vi "Experiment header-Interface module.vi"(4 "New Value":dbl, 6 "Name of parameter to update":string, 7 "Header file type":T7=enum."Params for funct acq w ROI or mscn", 8 "error in (no error)":errorcluster, 9 "All header parameters in":T1={"Imaging Protocol"=enum."AOL Z-Stack", "Number of POI"=0, "Number of Miniscans"=0, "Number of Trials"=0, "Number of Cycles "=0, "# Averaged Frames"=0, "Laser power (%)"=0, "Pockels"=0.0, "Acquisition Length (sec)"=0.0, "Fill time (us)"=0.0, "POI Dwell time (us)"=0.0, "Miniscan Dwell time per pixel (us)"=0.0, "PMT 1"=0.0, "PMT 2"=0.0, "Back Apperture"=0.0, "Zoom"=0.0, "Frame Size"=0, "Center Frequency"=0.0, "Field of View"=0.0, "DwellTime (us)"=0.0, "Wavelength (nm)"=0.0, "AOL Z"=0.0, "AOL Mode"=enum."Raster", "GridXY"=0.0, "GridZ"=0.0, "TriggerDelay (sec)"=0.0, "Number of Pixels in Miniscan"=0, "Experiment folder path"=path "", "X centre"=0.0, "Y centre"=0.0, "Angle (degrees)"=0.0, "Plane Mode"=0, "Software version"=0.0, "Objective"="Olympus  20X", "MotorZ Calibration"=0, "Pockels Calibration"=0, "Threshold"=[], "Video length (sec)"=0.0, "Frame rate (fps)"=0, "Rectangle ROI length (pixels)"=0, "Rectangle ROI height (pixels)"=0} {"Pockels" format="%#.6g"; "Software version" format="%#.6g"; "Plane Mode" items=["XY Plane"]; "Angle (degrees)" format="%#.6g"; "Frame Size" items=["100X100"=100, "128X128"=128, "200X200"=200, "256X256"=256, "512X512"=512, "1024x1024"=1024, "2048x2048"=2048]; "Back Apperture" format="%#.6g"; "PMT 2" format="%#.6g"; "PMT 1" format="%#.6g"; "Miniscan Dwell time per pixel (us)" format="%#.6g"; "Zoom" format="%#.6g"; "POI Dwell time (us)" format="%#.6g"; "Acquisition Length (sec)" format="%#.6g"; "Fill time (us)" format="%#.6g"}, 10 "Function":T8, 11 "Experiment data folder path":path) -> (0 "error out":errorcluster, 1 "All header parameters out":T1={"Imaging Protocol"=enum."AOL Z-Stack", "Number of POI"=0, "Number of Miniscans"=0, "Number of Trials"=0, "Number of Cycles "=0, "# Averaged Frames"=0, "Laser power (%)"=0, "Pockels"=0.0, "Acquisition Length (sec)"=0.0, "Fill time (us)"=0.0, "POI Dwell time (us)"=0.0, "Miniscan Dwell time per pixel (us)"=0.0, "PMT 1"=0.0, "PMT 2"=0.0, "Back Apperture"=0.0, "Zoom"=0.0, "Frame Size"=0, "Center Frequency"=0.0, "Field of View"=0.0, "DwellTime (us)"=0.0, "Wavelength (nm)"=0.0, "AOL Z"=0.0, "AOL Mode"=enum."Raster", "GridXY"=0.0, "GridZ"=0.0, "TriggerDelay (sec)"=0.0, "Number of Pixels in Miniscan"=0, "Experiment folder path"=path "", "X centre"=0.0, "Y centre"=0.0, "Angle (degrees)"=0.0, "Plane Mode"=0, "Software version"=0.0, "Objective"="Olympus  20X", "MotorZ Calibration"=0, "Pockels Calibration"=0, "Threshold"=[], "Video length (sec)"=0.0, "Frame rate (fps)"=0, "Rectangle ROI length (pixels)"=0, "Rectangle ROI height (pixels)"=0} {"Pockels" format="%#.6g"; "Software version" format="%#.6g"; "Plane Mode" items=["XY Plane"]; "Angle (degrees)" format="%#.6g"; "Frame Size" items=["100X100"=100, "128X128"=128, "200X200"=200, "256X256"=256, "512X512"=512, "1024x1024"=1024, "2048x2048"=2048]; "Back Apperture" format="%#.6g"; "PMT 2" format="%#.6g"; "PMT 1" format="%#.6g"; "Miniscan Dwell time per pixel (us)" format="%#.6g"; "Zoom" format="%#.6g"; "POI Dwell time (us)" format="%#.6g"; "Acquisition Length (sec)" format="%#.6g"; "Fill time (us)" format="%#.6g"})   [LabVIEW 2013]
uses:
  Typedefs/Header parameters cluster-ALL.ctl
  Typedefs/Imaging Protocols enum.ctl
  Typedefs/Frame Size.ctl
  Typedefs/AOL modes.ctl
  Typedefs/Plane Mode.ctl
  Typedefs/Objective selector control enum.ctl
  Typedefs/Header file interface module functions enum.ctl
  Typedefs/Header file type enum.ctl
  Typedefs/Save-Load-Save as-Load last enum.ctl
panel:
  in  "All params (internal)":T1={"Imaging Protocol"=enum."AOL Z-Stack", "Number of POI"=0, "Number of Miniscans"=0, "Number of Trials"=0, "Number of Cycles "=0, "# Averaged Frames"=0, "Laser power (%)"=0, "Pockels"=0.0, "Acquisition Length (sec)"=0.0, "Fill time (us)"=0.0, "POI Dwell time (us)"=0.0, "Miniscan Dwell time per pixel (us)"=0.0, "PMT 1"=0.0, "PMT 2"=0.0, "Back Apperture"=0.0, "Zoom"=0.0, "Frame Size"=0, "Center Frequency"=0.0, "Field of View"=0.0, "DwellTime (us)"=0.0, "Wavelength (nm)"=0.0, "AOL Z"=0.0, "AOL Mode"=enum."Raster", "GridXY"=0.0, "GridZ"=0.0, "TriggerDelay (sec)"=0.0, "Number of Pixels in Miniscan"=0, "Experiment folder path"=path "", "X centre"=0.0, "Y centre"=0.0, "Angle (degrees)"=0.0, "Plane Mode"=0, "Software version"=0.0, "Objective"="Olympus  20X", "MotorZ Calibration"=0, "Pockels Calibration"=0, "Threshold"=[], "Video length (sec)"=0.0, "Frame rate (fps)"=0, "Rectangle ROI length (pixels)"=0, "Rectangle ROI height (pixels)"=0} {"Pockels" format="%#.6g"; "Software version" format="%#.6g"; "Plane Mode" items=["XY Plane"]; "Angle (degrees)" format="%#.6g"; "Frame Size" items=["100X100"=100, "128X128"=128, "200X200"=200, "256X256"=256, "512X512"=512, "1024x1024"=1024, "2048x2048"=2048]; "Back Apperture" format="%#.6g"; "PMT 2" format="%#.6g"; "PMT 1" format="%#.6g"; "Miniscan Dwell time per pixel (us)" format="%#.6g"; "Zoom" format="%#.6g"; "POI Dwell time (us)" format="%#.6g"; "Acquisition Length (sec)" format="%#.6g"; "Fill time (us)" format="%#.6g"}
  # "Used with the \"Update specific value in memory\" function only"
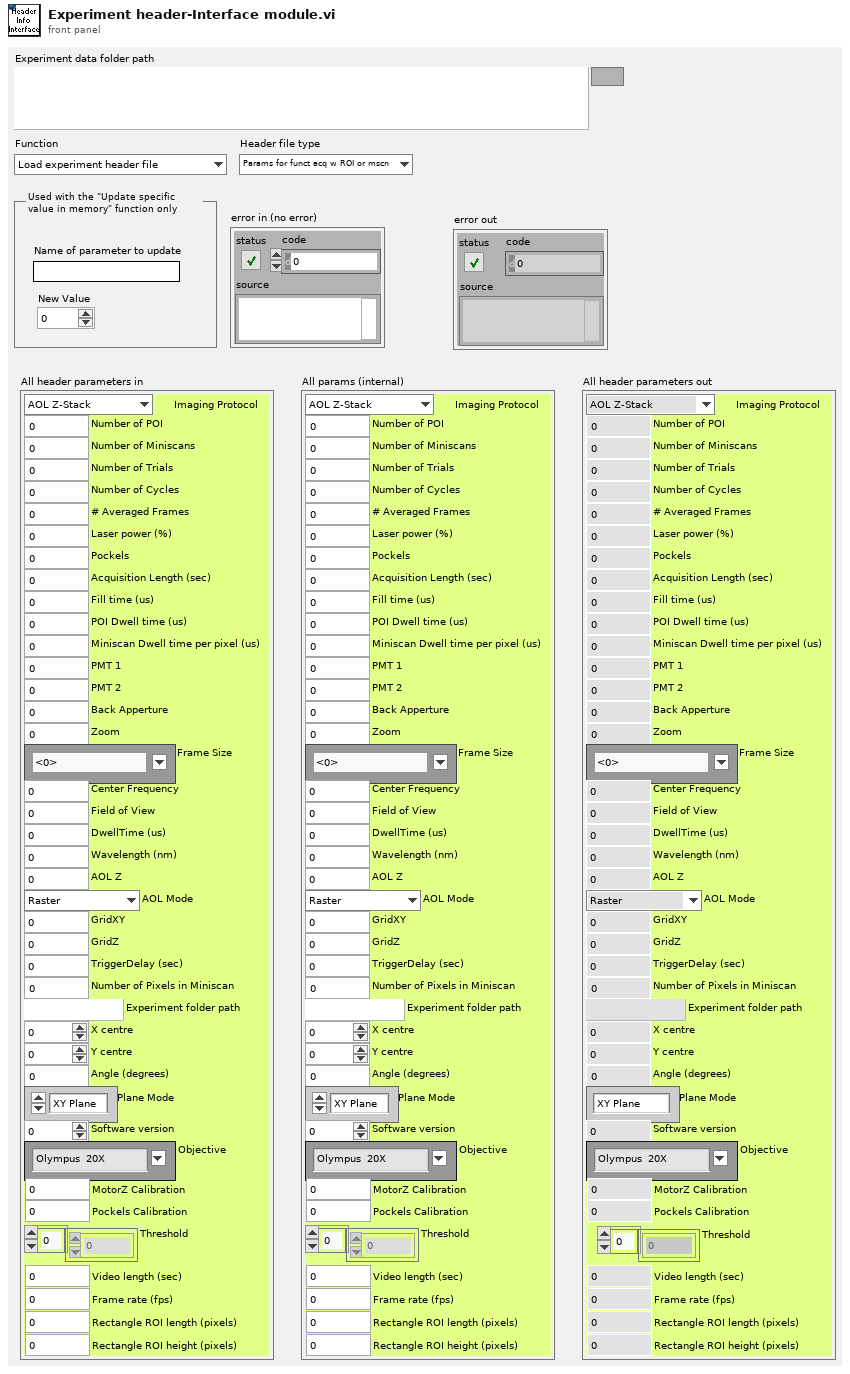
[diagram p1: front panel]
types:
  T1 = typedef "Header parameters cluster-ALL.ctl" = cluster{"Imaging Protocol":T2, "Number of POI":u16, "Number of Miniscans":u16, "Number of Trials":u16, "Number of Cycles ":u64, "# Averaged Frames":u16, "Laser power (%)":u8, "Pockels":dbl, "Acquisition Length (sec)":dbl, "Fill time (us)":dbl, "POI Dwell time (us)":dbl, "Miniscan Dwell time per pixel (us)":dbl, "PMT 1":dbl, "PMT 2":dbl, "Back Apperture":dbl, "Zoom":dbl, "Frame Size":T3, "Center Frequency":dbl, "Field of View":dbl, "DwellTime (us)":dbl, "Wavelength (nm)":dbl, "AOL Z":dbl, "AOL Mode":T4, "GridXY":dbl, "GridZ":dbl, "TriggerDelay (sec)":dbl, "Number of Pixels in Miniscan":u16, "Experiment folder path":path, "X centre":dbl, "Y centre":dbl, "Angle (degrees)":dbl, "Plane Mode":T5, "Software version":dbl, "Objective":T6, "MotorZ Calibration":u32, "Pockels Calibration":u32, "Threshold":u16[], "Video length (sec)":dbl, "Frame rate (fps)":u8, "Rectangle ROI length (pixels)":u16, "Rectangle ROI height (pixels)":u16}
  T2 = typedef "Imaging Protocols enum.ctl" = enum16{"AOL Z-Stack", "Motor Z Stack", "Functional Acquisition", "Single Plane Acquisition", "Volume Acquisition", "Live Imaging", "Live Plane Imaging", "Live Volume Imaging"}
  T3 = typedef "Frame Size.ctl" = u16
  T4 = typedef "AOL modes.ctl" = enum16{"Raster", "Structural", "Pointing", "Mini Scan", "Alignment"}
  T5 = typedef "Plane Mode.ctl" = u16
  T6 = typedef "Objective selector control enum.ctl" = string
  T7 = typedef "Header file type enum.ctl" = enum16{"All parameters", "Params for funct acq w ROI or mscn", "Params for funct acq w rectangles", "Live imaging header parameters", "AOL Parameters"}
  T8 = typedef "Header file interface module functions enum.ctl" = enum16{"Load experiment header file", "Save experiment header file", "Clear stored values", "Read stored values", "Update specific value in memory", "Update all values in memory"}
  T9 = typedef "Save-Load-Save as-Load last enum.ctl" = enum16{"Save file", "Save file as", "Load file", "Load last file"}
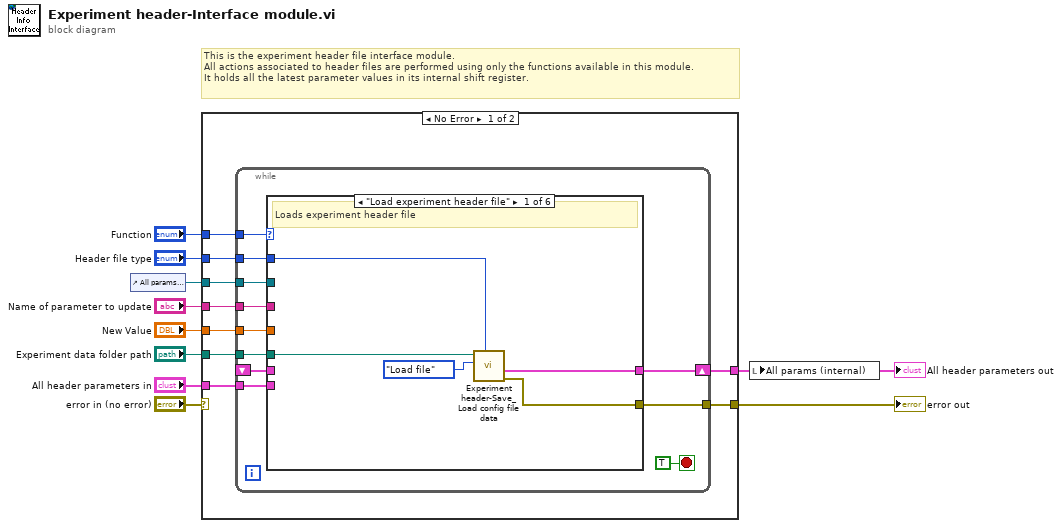
[diagram p0: block diagram]
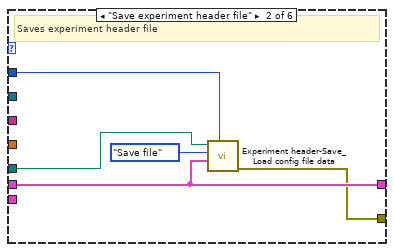
[diagram p2: hidden frame]
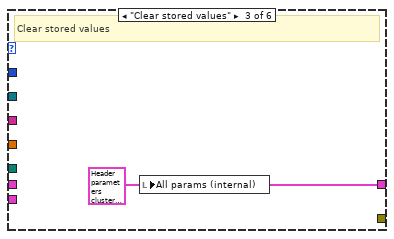
[diagram p3: hidden frame]
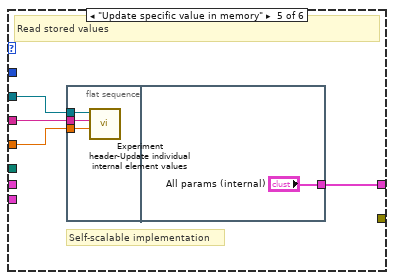
[diagram p5: hidden frame]
diagram:
  # "This is the experiment header file interface module.\nAll actions associated to header files are performed using only the functions available in this module.\nIt holds all the latest parameter values in its internal shift register."
  n1 = control-ref of="All params (internal)"() -> (w2:refnum<vi>)
  n2 = case shown="No Error" "error in (no error)" {
    selector: "error in (no error)" -> [_ w52]
    tunnel: [w19 _] -> w1
    tunnel: "Function" -> [w18 _]
    tunnel: "Name of parameter to update" -> [w17 _]
    tunnel: "New Value" -> [w16 _]
    tunnel: "Experiment data folder path" -> [w15 _]
    tunnel: [w14 w52] -> w8
    tunnel: "All header parameters in" -> [w13 _]
    tunnel: "Header file type" -> [w12 _]
    tunnel: w2 -> [w11 _]
    frame No Error {
      n3 = while {
        shift-right: [w29] -> w19
        shift-left: _ -> [w27]
        tunnel: w18 -> [w28]
        tunnel: w17 -> [w26]
        tunnel: w16 -> [w25]
        tunnel: w15 -> [w23]
        tunnel: [w24] -> w14
        tunnel: w13 -> [w22]
        tunnel: w12 -> [w21]
        tunnel: w11 -> [w20]
        stop <- TRUE stop-if-true
        n4 = case shown="\"Load experiment header file\"" w28 {
          tunnel: [w31 w38 w41 w42 w44 w51] -> w29
          tunnel: w27 -> [_ w38 _ w42 _ _]
          tunnel: w26 -> [_ _ _ _ w46 _]
          tunnel: w25 -> [_ _ _ _ w45 _]
          tunnel: [w34 w36 _ _ _ _] -> w24
          tunnel: w23 -> [w35 w39 _ _ _ _]
          tunnel: w22 -> [_ _ _ _ _ w51]
          tunnel: w21 -> [w32 w37 _ _ _ _]
          tunnel: w20 -> [_ _ _ _ w43 _]
          frame "Load experiment header file" {
            # "Loads experiment header file"
            n5 = call "Experiment header-Save_Load config file data.vi"("Header file type"=w32, "Function"=Save-Load-Save_as-Load_last_enum."Load file", "Experiment data folder path"=w35) -> ("error out"=w34:errorcluster, "All header parameters out"=w31:T1)  [unwired: 7 in]
          }
          frame "Save experiment header file" {
            # "Saves experiment header file"
            n6 = call "Experiment header-Save_Load config file data.vi"("Header file type"=w37, "All header parameters in"=w38, "Function"=Save-Load-Save_as-Load_last_enum."Save file", "Experiment data folder path"=w39) -> ("error out"=w36:errorcluster)  [unwired: 6 in, 1 out]
          }
          frame "Clear stored values" {
            w41 = T1 {"Imaging Protocol"=enum."AOL Z-Stack", "Number of POI"=0, "Number of Miniscans"=0, "Number of Trials"=0, "Number of Cycles "=0, "# Averaged Frames"=0, "Laser power (%)"=0, "Pockels"=0.0, "Acquisition Length (sec)"=0.0, "Fill time (us)"=0.0, "POI Dwell time (us)"=0.0, "Miniscan Dwell time per pixel (us)"=0.0, "PMT 1"=0.0, "PMT 2"=0.0, "Back Apperture"=0.0, "Zoom"=0.0, "Frame Size"=0, "Center Frequency"=0.0, "Field of View"=0.0, "DwellTime (us)"=0.0, "Wavelength (nm)"=0.0, "AOL Z"=0.0, "AOL Mode"=enum."Raster", "GridXY"=0.0, "GridZ"=0.0, "TriggerDelay (sec)"=0.0, "Number of Pixels in Miniscan"=0, "Experiment folder path"=path "", "X centre"=0.0, "Y centre"=0.0, "Angle (degrees)"=0.0, "Plane Mode"=0, "Software version"=0.0, "Objective"="", "MotorZ Calibration"=0, "Pockels Calibration"=0, "Threshold"=[], "Video length (sec)"=0.0, "Frame rate (fps)"=0, "Rectangle ROI length (pixels)"=0, "Rectangle ROI height (pixels)"=0} ("All header parameters in")
            # "Clear stored values"
            n7 = local write "All params (internal)"(w41) -> ()
          }
          frame "Read stored values", Default {
            # "Read stored values"
          }
          frame "Update specific value in memory" {
            # "Self-scalable implementation"
            # "Read stored values"
            n8 = flat-sequence {
              tunnel: w43 -> [w47]
              tunnel: w46 -> [w49]
              tunnel: w45 -> [w48]
              tunnel: ["All params (internal)"] -> w44
              frame #0 {
                n9 = call "Experiment header-Update individual internal element values.vi"("Value"=w48, "Name of parameter to update"=w49, "All params (internal)"=w47) -> ()  [unwired: 9 in]
              }
              frame #1 {
              }
            }
          }
          frame "Update all values in memory" {
            # "Read stored values"
          }
        }
      }
    }
    frame Error {
    }
  }
  "All header parameters out" <- w1
  "error out" <- w8
  n10 = local write "All params (internal)"(w1) -> ()
